vi "Part 2.vi"(11 "Input":string) -> (3 "Output":i64)   [LabVIEW 2021]
uses:
  <userlib>/_OpenG.lib/string/string.llb/Convert EOLs (String)__ogtk.vi
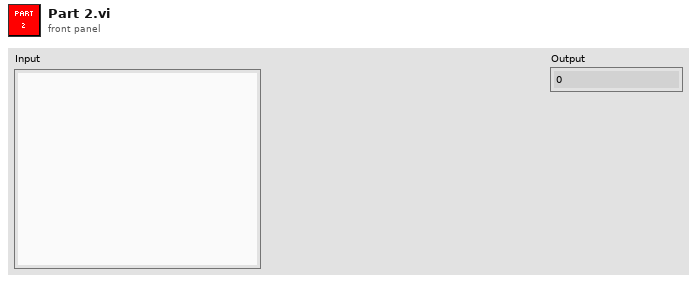
[diagram p1: front panel]
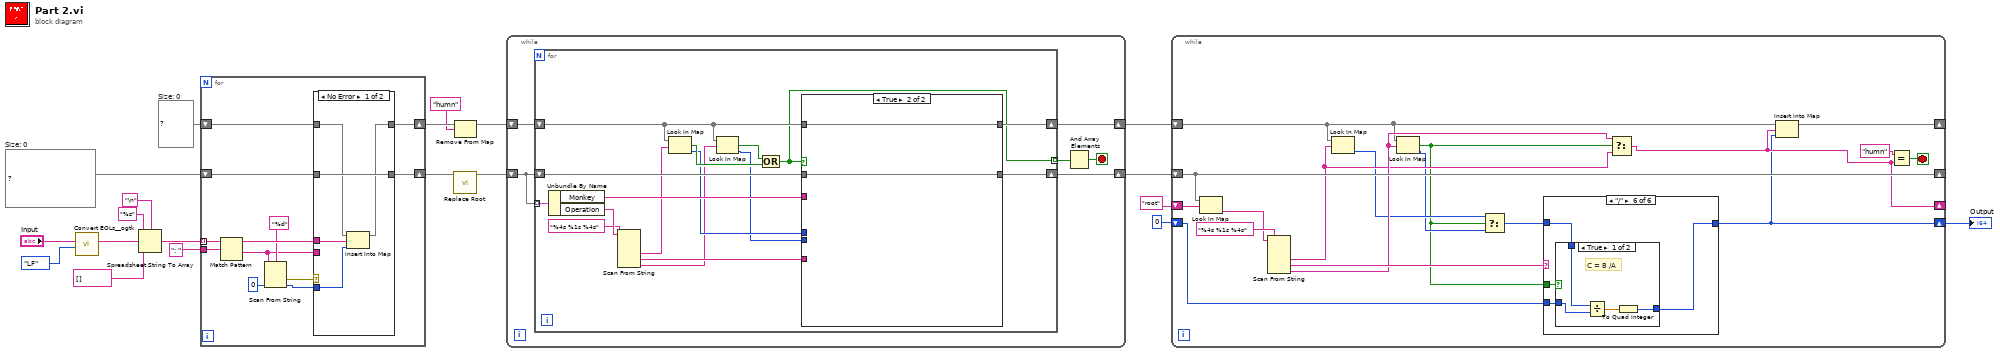
[diagram p0: block diagram]
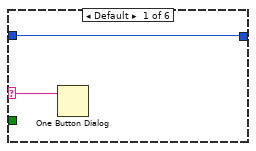
[diagram p2: hidden frame]
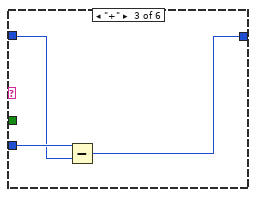
[diagram p4: hidden frame]
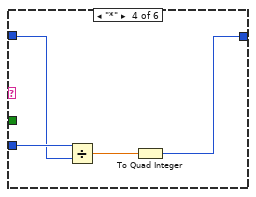
[diagram p5: hidden frame]
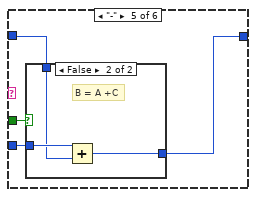
[diagram p6: hidden frame]
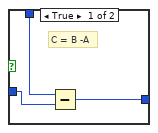
[diagram p7: hidden frame]
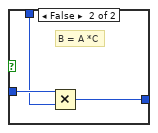
[diagram p8: hidden frame]
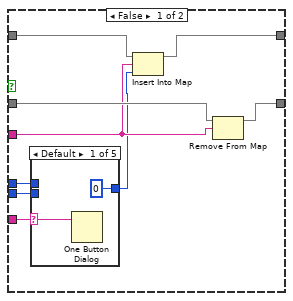
[diagram p9: hidden frame]
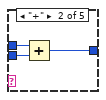
[diagram p10: hidden frame]
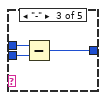
[diagram p11: hidden frame]
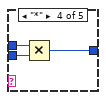
[diagram p12: hidden frame]
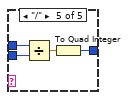
[diagram p13: hidden frame]
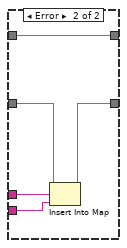
[diagram p14: hidden frame]
diagram:
  w11 = map{string, i64} {}  # Size: 0
  w12 = map{string, string} {}  # Size: 0
  n1 = call-poly <userlib>:"Convert EOLs__ogtk.vi"("Convert to:"=enum16{"CR", "LF", "CRLF"}."LF", "String in"="Input") -> ("String out"=w16:string)  [unwired: 9 in]
  n2 = Spreadsheet String To Array(delimiter (Tab)="\n", format string="%s", spreadsheet string=w16, array type (2D Dbl)=string[] []) -> (array=w14:string[])
  n3 = for {
    tunnel: w14 -> [w32] mode=indexing
    shift-right: [w28] -> w4
    shift-left: w12 -> [w29]
    tunnel: ": " -> [w31]
    shift-right: [w23] -> w10
    shift-left: w11 -> [w24]
    n4 = Match Pattern(string=w32, regular expression=w31) -> (before substring=w30:string, after substring=w21:string)  [unwired: 1 in, 2 out]
    n5 = Scan From String(format string="%d", input string=w21, default 1=i64 0 ("default value 1")) -> (error out=w25:errorcluster, output 1=w22:i64)  [unwired: 2 in, 2 out]
    n6 = case shown="No Error" w25 {
      tunnel: w30 -> [w36 w42]
      tunnel: w29 -> [w37 w41]
      tunnel: [w37 w40] -> w28
      tunnel: w24 -> [w35 w39]
      tunnel: [w34 w39] -> w23
      tunnel: w22 -> [w33 _]
      tunnel: w21 -> [_ w38]
      frame No Error {
        n7 = Insert Into Map(map in=w35, key=w36, value=w33) -> (map out=w34:map{string, i64})  [unwired: 2 out]
      }
      frame Error {
        n8 = Insert Into Map(map in=w41, key=w42, value=w38) -> (map out=w40:map{string, string})  [unwired: 2 out]
      }
    }
  }
  n9 = call "Replace Root.vi"("Map in"=w4) -> ("Map out"=w3:map{string, string})  [unwired: 10 in]
  n10 = Remove From Map(10:"humn" ("key"), 11:w10) -> (3:w9:map{string, i64})  [unwired: 2 out]
  n11 = while {
    shift-right: [w47] -> w7
    shift-left: w9 -> [w48]
    shift-right: [w45] -> w6
    shift-left: w3 -> [w46]
    stop <- w43 stop-if-true
    n12 = for {
      tunnel: w46 -> [w61] mode=indexing
      shift-right: [w62] -> w47
      shift-left: w48 -> [w57]
      shift-right: [w63] -> w45
      shift-left: w46 -> [w64]
      tunnel: [w50] -> w44 mode=indexing
      n13 = Unbundle By Name(w61) -> ("Monkey"=w60:string, "Operation"=w59:string)
      n14 = Scan From String(format string="%4s %1s %4s", input string=w59) -> (output 1=w52:string, output 2=w55:string, output 3=w51:string)  [unwired: 5 in, 3 out]
      n15 = Look In Map(map=w57, key=w52) -> (key not found?=w56:bool, value=w54:i64)  [unwired: 1 in]
      n16 = Look In Map(map=w57, key=w51) -> (key not found?=w49:bool, value=w53:i64)  [unwired: 1 in]
      n17 = Compound Arithmetic op=OR(w49, w56) -> (w50:bool)
      n18 = case shown="True" w50 {
        tunnel: w64 -> [w72 w89]
        tunnel: [w73 w89] -> w63
        tunnel: w57 -> [w70 w90]
        tunnel: [w71 w90] -> w62
        tunnel: w60 -> [w69 _]
        tunnel: w55 -> [w68 _]
        tunnel: w54 -> [w67 _]
        tunnel: w53 -> [w66 _]
        frame False {
          n19 = case shown="Default" w68 {
            selector: w68 -> [w74 _ _ _ _]
            tunnel: w67 -> [_ w78 w81 w84 w88]
            tunnel: w66 -> [_ w77 w80 w83 w87]
            tunnel: [i64 0 w76 w79 w82 w85] -> w65
            frame Default {
              n20 = One Button Dialog(message=w74) -> ()  [unwired: 1 in, 1 out]
            }
            frame "+" {
              n21 = Add(x=w78, y=w77) -> (x+y=w76:i64)
            }
            frame "-" {
              n22 = Subtract(x=w81, y=w80) -> (x-y=w79:i64)
            }
            frame "*" {
              n23 = Multiply(x=w84, y=w83) -> (x*y=w82:i64)
            }
            frame "/" {
              n24 = Divide(x=w88, y=w87) -> (x/y=w86:dbl)
              n25 = To Quad Integer(1:w86) -> (0:w85:i64)
            }
          }
          n26 = Insert Into Map(map in=w70, key=w69, value=w65) -> (map out=w71:map{string, i64})  [unwired: 2 out]
          n27 = Remove From Map(10:w69, 11:w72) -> (3:w73:map{string, string})  [unwired: 2 out]
        }
        frame True {
        }
      }
    }
    n28 = And Array Elements(Boolean array=w44) -> (logical AND=w43:bool)
  }
  n29 = while {
    shift-right: [w95] -> _
    shift-left: w7 -> [w96]
    shift-right: [w105] -> _
    shift-left: w6 -> [w105]
    shift-right: [w94] -> _
    shift-left: "root" -> [w108]
    shift-right: [w93] -> w1
    shift-left: i64 0 -> [w92]
    stop <- w103 stop-if-true
    n30 = Look In Map(map=w105, key=w108) -> (value=w106:string)  [unwired: 1 in, 1 out]
    n31 = Scan From String(format string="%4s %1s %4s", input string=w106) -> (output 1=w100:string, output 2=w104:string, output 3=w101:string)  [unwired: 5 in, 3 out]
    n32 = Look In Map(map=w96, key=w100) -> (value=w99:i64)  [unwired: 1 in, 1 out]
    n33 = Look In Map(map=w96, key=w101) -> (key not found?=w91:bool, value=w98:i64)  [unwired: 1 in]
    n34 = Select(t=w99, s=w91, f=w98) -> (s? t:f=w97:i64)
    n35 = case shown="\"/\"" w104 {
      selector: w104 -> [w110 _ _ _ _ _]
      tunnel: w97 -> [w109 w111 w112 w116 w120 w130]
      tunnel: [w109 w111 w113 w115 w121 w131] -> w93
      tunnel: w92 -> [_ _ w114 w118 w122 w132]
      tunnel: w91 -> [_ _ _ _ w119 w129]
      frame Default {
        n36 = One Button Dialog(message=w110) -> ()  [unwired: 1 in, 1 out]
      }
      frame "=" {
      }
      frame "+" {
        n37 = Subtract(x=w114, y=w112) -> (x-y=w113:i64)
      }
      frame "*" {
        n38 = Divide(x=w118, y=w116) -> (x/y=w117:dbl)
        n39 = To Quad Integer(1:w117) -> (0:w115:i64)
      }
      frame "-" {
        n40 = case shown="False" w119 {
          tunnel: w122 -> [w123 w128]
          tunnel: [w125 w127] -> w121
          tunnel: w120 -> [w124 w126]
          frame True {
            # "C = B -A"
            n41 = Subtract(x=w124, y=w123) -> (x-y=w125:i64)
          }
          frame False {
            # "B = A +C"
            n42 = Add(x=w128, y=w126) -> (x+y=w127:i64)
          }
        }
      }
      frame "/" {
        n43 = case shown="True" w129 {
          tunnel: w132 -> [w134 w139]
          tunnel: [w133 w138] -> w131
          tunnel: w130 -> [w135 w137]
          frame True {
            # "C = B /A"
            n44 = Divide(x=w135, y=w134) -> (x/y=w136:dbl)
            n45 = To Quad Integer(1:w136) -> (0:w133:i64)
          }
          frame False {
            # "B = A *C"
            n46 = Multiply(x=w139, y=w137) -> (x*y=w138:i64)
          }
        }
      }
    }
    n47 = Select(t=w101, s=w91, f=w100) -> (s? t:f=w94:string)
    n48 = Insert Into Map(map in=w96, key=w94, value=w93) -> (map out=w95:map{string, i64})  [unwired: 2 out]
    n49 = Equal?(x="humn", y=w94) -> (x = y?=w103:bool)
  }
  "Output" <- w1
